vi "Finish.vi"   [LabVIEW 2017]
doc: "This VI is called just before exiting. It is expected to close I/O refnum, save collected data, etc."
uses:
  <vilib>/Rock Robotics/WPI/Utilities/WPI_GetSetVariantRefNum.vi
  <vilib>/Rock Robotics/WPI/Ultrasonic/WPI_SonarSRF04DigitalRefNum Registry Get.vi
  <vilib>/Rock Robotics/WPI/Ultrasonic/WPI_SonarSRF04DigitalClose.vi
types:
  T1 = typedef "WPI_UltrasonicDeviceRef.ctl" = cluster{"DevStatus":errorcluster, "Ping Channel":T2, "Echo Channel":T2, "CntIndex":T3}
  T2 = typedef "FPGA_DIOChannel.ctl" = enum8{"DIO 0", "DIO 1", "DIO 2", "DIO 3", "DIO 4", "DIO 5", "DIO 6", "DIO 7", "DIO 8", "DIO 9", "DIO MXP 0", "DIO MXP 1", "DIO MXP 2", "DIO MXP 3", "DIO MXP 4", "DIO MXP 5", "DIO MXP 6", "DIO MXP 7", "DIO MXP 8", "DIO MXP 9", "DIO MXP 10", "DIO MXP 11", "DIO MXP 12", "DIO MXP 13", "DIO MXP 14", "DIO MXP 15", "SPI Port CS1", "SPI Port CS2", "SPI Port CS3", "SPI Port MISO", "SPI Port MOSI", "Invalid"}
  T3 = typedef "FPGA_CounterCtrSystemIndex.ctl" = enum8{"Ctr 0", "Ctr 1", "Ctr 2", "Ctr 3", "Ctr 4", "Ctr 5", "Ctr 6", "Ctr 7", "Invalid"}
  T4 = typedef "WPI_SwitchDevRef.ctl" = cluster{"DevStatus":errorcluster, "DIO Channel":T2, "CntIndex":T3, "Normally Closed":bool}
  T5 = typedef "WPI_MotorControlDeviceRef.ctl" = cluster{"DeviceStatus":errorcluster, "Type":T6, "PWM":cluster{"PWM Channel":T7, "DeadBand":T8}, "CAN":cluster{"Device Number":u8, "SetOutput VI Ref":variant, "GetOutput VI Ref":variant, "Enable VI Ref":variant, "Disable VI Ref":variant, "Data":variant}, "Invert":bool, "DIO PWM":cluster{"PWM \"Enable\" Channel":T7, "DIOChannel":T2, "PWM Rate":dbl}}
  T6 = typedef "WPI_MotorControlType.ctl" = enum16{"PWM", "CAN", "DIO PWM"}
  T7 = typedef "FPGA_DIOPWMChannel.ctl" = enum8{"PWM 0", "PWM 1", "PWM 2", "PWM 3", "PWM 4", "PWM 5", "PWM 6", "PWM 7", "PWM 8", "PWM 9", "PWM MXP 0", "PWM MXP 1", "PWM MXP 2", "PWM MXP 3", "PWM MXP 4", "PWM MXP 5", "PWM MXP 6", "PWM MXP 7", "PWM MXP 8", "PWM MXP 9", "Invalid"}
  T8 = typedef "WPI_PWMDeadband.ctl" = cluster{"Name":string, "maxPositivePwm":i32, "minPositivePwm":i32, "centerPwm":i32, "maxNegativePwm":i32, "minNegativePwm":i32, "angularRange":u16}
  T9 = typedef "WPI_SolenoidDevRef.ctl" = cluster{"DevStatus":errorcluster, "Pneumatics Control Module":u8, "Forward Solenoid Channel":T10, "Reverse Solenoid Channel":T10}
  T10 = typedef "WPI_SolenoidChannel.ctl" = enum8{"Solenoid 0", "Solenoid 1", "Solenoid 2", "Solenoid 3", "Solenoid 4", "Solenoid 5", "Solenoid 6", "Solenoid 7", "Invalid"}
  T11 = typedef "WPI_JoystickDevRef.ctl" = cluster{"Device":T12}
  T12 = typedef "WPI_JoystickDeviceEnum.ctl" = enum16{"USB 0", "USB 1", "USB 2", "USB 3", "USB 4", "USB 5"}
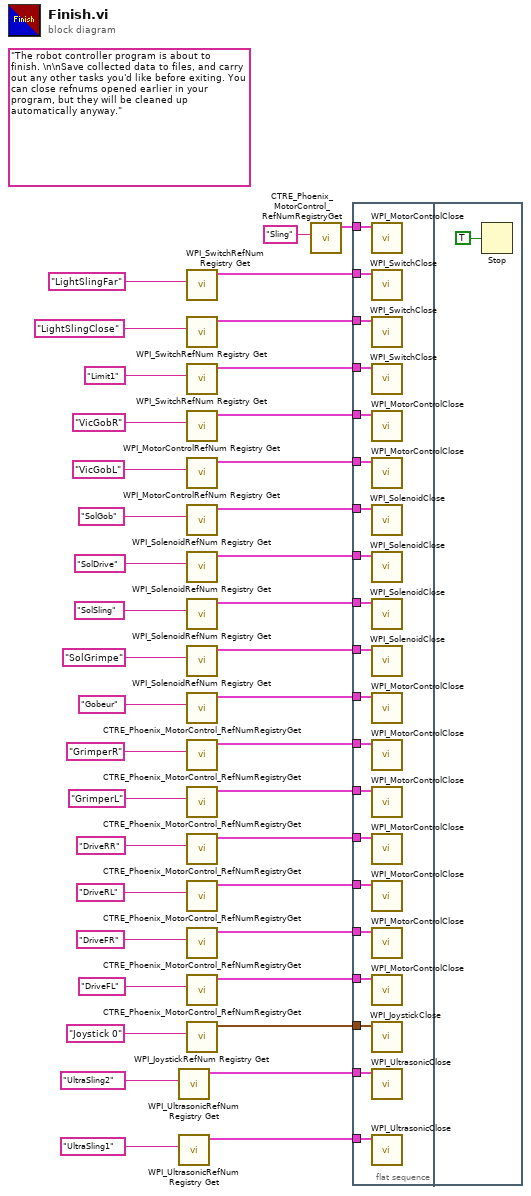
[diagram p0: block diagram]
diagram:
  (unwired) "The robot controller program is about to finish. \n\nSave collected data to files, and carry out any other tasks you'd like before exiting. You can close refnums opened earlier in your program, but they will be cleaned up automatically anyway."
  n1 = call-poly <vilib>:"WPI_UltrasonicRefNum Registry Get.vi"("refnum name"="UltraSling2") -> ("SonarSRF04DevRef"=w19:T1)  [unwired: 9 in, 1 out]
  n2 = call-poly <vilib>:"WPI_UltrasonicRefNum Registry Get.vi"("refnum name"="UltraSling1") -> ("SonarSRF04DevRef"=w22:T1)  [unwired: 9 in, 1 out]
  n3 = call <vilib>:"WPI_SwitchRefNum Registry Get.vi"("refnum name"="LightSlingFar") -> ("SwitchDevRef"=w16:T4)  [unwired: 9 in, 1 out]
  n4 = call <vilib>:"WPI_SwitchRefNum Registry Get.vi"("refnum name"="LightSlingClose") -> ("SwitchDevRef"=w17:T4)  [unwired: 9 in, 1 out]
  n5 = call <vilib>:"WPI_SwitchRefNum Registry Get.vi"("refnum name"="Limit1") -> ("SwitchDevRef"=w18:T4)  [unwired: 9 in, 1 out]
  n6 = call <vilib>:"WPI_MotorControlRefNum Registry Get.vi"("refnum name"="VicGobR") -> ("MotorControlDevRef"=w3:T5)  [unwired: 9 in, 1 out]
  n7 = call <vilib>:"WPI_MotorControlRefNum Registry Get.vi"("refnum name"="VicGobL") -> ("MotorControlDevRef"=w4:T5)  [unwired: 9 in, 1 out]
  n8 = call <vilib>:"WPI_SolenoidRefNum Registry Get.vi"("refnum name"="SolGob") -> ("SolenoidDevRef"=w9:T9)  [unwired: 9 in, 1 out]
  n9 = call <vilib>:"WPI_SolenoidRefNum Registry Get.vi"("refnum name"="SolDrive") -> ("SolenoidDevRef"=w10:T9)  [unwired: 9 in, 1 out]
  n10 = call <vilib>:"WPI_SolenoidRefNum Registry Get.vi"("refnum name"="SolSling") -> ("SolenoidDevRef"=w11:T9)  [unwired: 9 in, 1 out]
  n11 = call <vilib>:"WPI_SolenoidRefNum Registry Get.vi"("refnum name"="SolGrimpe") -> ("SolenoidDevRef"=w12:T9)  [unwired: 9 in, 1 out]
  n12 = call "CTRE_Phoenix_MotorControl_RefNumRegistryGet.vi"("refnum name"="Gobeur") -> ("PhoenixMotorControlDevRef"=w23:T5)  [unwired: 9 in, 1 out]
  n13 = call "CTRE_Phoenix_MotorControl_RefNumRegistryGet.vi"("refnum name"="GrimperR") -> ("PhoenixMotorControlDevRef"=w24:T5)  [unwired: 9 in, 1 out]
  n14 = call "CTRE_Phoenix_MotorControl_RefNumRegistryGet.vi"("refnum name"="GrimperL") -> ("PhoenixMotorControlDevRef"=w25:T5)  [unwired: 9 in, 1 out]
  n15 = call "CTRE_Phoenix_MotorControl_RefNumRegistryGet.vi"("refnum name"="DriveRR") -> ("PhoenixMotorControlDevRef"=w27:T5)  [unwired: 9 in, 1 out]
  n16 = call "CTRE_Phoenix_MotorControl_RefNumRegistryGet.vi"("refnum name"="DriveRL") -> ("PhoenixMotorControlDevRef"=w28:T5)  [unwired: 9 in, 1 out]
  n17 = call "CTRE_Phoenix_MotorControl_RefNumRegistryGet.vi"("refnum name"="DriveFR") -> ("PhoenixMotorControlDevRef"=w29:T5)  [unwired: 9 in, 1 out]
  n18 = call "CTRE_Phoenix_MotorControl_RefNumRegistryGet.vi"("refnum name"="DriveFL") -> ("PhoenixMotorControlDevRef"=w38:T5)  [unwired: 9 in, 1 out]
  n19 = call <vilib>:"WPI_JoystickRefNum Registry Get.vi"("refnum name"="Joystick 0") -> ("JoystickDevRef"=w39:T11)  [unwired: 1 in, 9 out]
  n20 = call "CTRE_Phoenix_MotorControl_RefNumRegistryGet.vi"("refnum name"="Sling") -> ("PhoenixMotorControlDevRef"=w26:T5)  [unwired: 9 in, 1 out]
  n21 = flat-sequence {
    tunnel: w39 -> [w60]
    tunnel: w38 -> [w59]
    tunnel: w29 -> [w58]
    tunnel: w28 -> [w57]
    tunnel: w27 -> [w56]
    tunnel: w26 -> [w55]
    tunnel: w25 -> [w54]
    tunnel: w24 -> [w53]
    tunnel: w23 -> [w52]
    tunnel: w22 -> [w51]
    tunnel: w19 -> [w50]
    tunnel: w18 -> [w49]
    tunnel: w17 -> [w48]
    tunnel: w16 -> [w47]
    tunnel: w12 -> [w46]
    tunnel: w11 -> [w45]
    tunnel: w10 -> [w44]
    tunnel: w9 -> [w43]
    tunnel: w4 -> [w42]
    tunnel: w3 -> [w41]
    frame #0 {
      n22 = call <vilib>:"WPI_MotorControlClose.vi"("MotorControlDevRef"=w55) -> ()  [unwired: 10 in, 1 out]
      n23 = call <vilib>:"WPI_SwitchClose.vi"("SwitchDevRef"=w47) -> ()  [unwired: 10 in, 1 out]
      n24 = call <vilib>:"WPI_SwitchClose.vi"("SwitchDevRef"=w48) -> ()  [unwired: 10 in, 1 out]
      n25 = call <vilib>:"WPI_SwitchClose.vi"("SwitchDevRef"=w49) -> ()  [unwired: 10 in, 1 out]
      n26 = call <vilib>:"WPI_MotorControlClose.vi"("MotorControlDevRef"=w41) -> ()  [unwired: 10 in, 1 out]
      n27 = call <vilib>:"WPI_MotorControlClose.vi"("MotorControlDevRef"=w42) -> ()  [unwired: 10 in, 1 out]
      n28 = call <vilib>:"WPI_SolenoidClose.vi"("SolenoidDevRef"=w43) -> ()  [unwired: 10 in, 1 out]
      n29 = call <vilib>:"WPI_SolenoidClose.vi"("SolenoidDevRef"=w44) -> ()  [unwired: 10 in, 1 out]
      n30 = call <vilib>:"WPI_SolenoidClose.vi"("SolenoidDevRef"=w45) -> ()  [unwired: 10 in, 1 out]
      n31 = call <vilib>:"WPI_SolenoidClose.vi"("SolenoidDevRef"=w46) -> ()  [unwired: 10 in, 1 out]
      n32 = call <vilib>:"WPI_MotorControlClose.vi"("MotorControlDevRef"=w52) -> ()  [unwired: 10 in, 1 out]
      n33 = call <vilib>:"WPI_MotorControlClose.vi"("MotorControlDevRef"=w53) -> ()  [unwired: 10 in, 1 out]
      n34 = call <vilib>:"WPI_MotorControlClose.vi"("MotorControlDevRef"=w54) -> ()  [unwired: 10 in, 1 out]
      n35 = call <vilib>:"WPI_MotorControlClose.vi"("MotorControlDevRef"=w56) -> ()  [unwired: 10 in, 1 out]
      n36 = call <vilib>:"WPI_MotorControlClose.vi"("MotorControlDevRef"=w57) -> ()  [unwired: 10 in, 1 out]
      n37 = call <vilib>:"WPI_MotorControlClose.vi"("MotorControlDevRef"=w58) -> ()  [unwired: 10 in, 1 out]
      n38 = call <vilib>:"WPI_MotorControlClose.vi"("MotorControlDevRef"=w59) -> ()  [unwired: 10 in, 1 out]
      n39 = call <vilib>:"WPI_JoystickClose.vi"("JoystickDevRef"=w60) -> ()  [unwired: 11 out]
      n40 = call-poly <vilib>:"WPI_UltrasonicClose.vi"("SonarSRF04DevRef"=w50) -> ()  [unwired: 10 in, 1 out]
      n41 = call-poly <vilib>:"WPI_UltrasonicClose.vi"("SonarSRF04DevRef"=w51) -> ()  [unwired: 10 in, 1 out]
    }
    frame #1 {
      n42 = Stop(stop? (T)=TRUE ("Quit")) -> ()
    }
  }
